vi "Channel_OFFSet.vi"(7 "Write?":bool, 8 "Error":errorcluster caption="错误输入（无错误）", 9 "Offset":dbl, 10 "Channel":u32, 11 "VISA resource name":refnum<visa-resource-name>) -> (0 "Error out":errorcluster, 2 "Offset out":dbl, 3 "VISA resource name out":refnum<visa-resource-name>)   [LabVIEW 2020]
doc: "屏幕中心显示的值"
panel:
  out "读取缓冲区":string
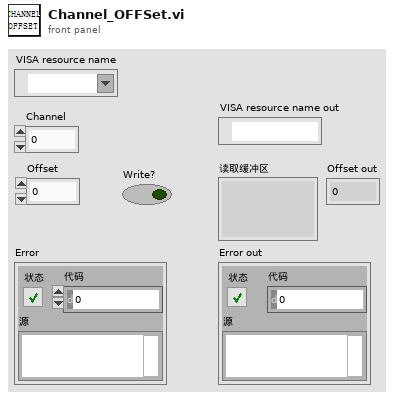
[diagram p1: front panel]
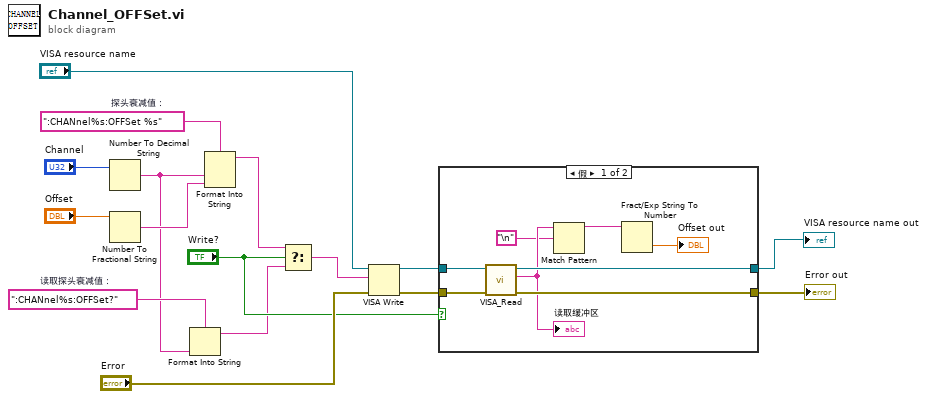
[diagram p0: block diagram]
diagram:
  w5 = ":CHANnel%s:OFFSet?"  # 读取探头衰减值：
  w9 = ":CHANnel%s:OFFSet %s"  # 探头衰减值：
  n1 = Number To Decimal String(number="Channel") -> (decimal integer string=w4:string)  [unwired: 1 in]
  n2 = Number To Fractional String(number="Offset") -> (F-format string=w7:string)  [unwired: 3 in]
  n3 = Format Into String(format string=w5, w4) -> (resulting string=w3:string)  [unwired: 2 in, 1 out]
  n4 = Format Into String(format string=w9, w4, w7) -> (resulting string=w6:string)  [unwired: 2 in, 1 out]
  n5 = Select(t=w6, s="Write?", f=w3) -> (s? t:f=w14:string)
  n6 = VISA Write(VISA resource name="VISA resource name", write buffer=w14, error in (no error)="Error") -> (VISA resource name out=w10:refnum<visa-resource-name>, error out=w12:errorcluster)  [unwired: 1 out]
  n7 = case shown="假" "Write?" {
    tunnel: w10 -> [w24 w26]
    tunnel: w12 -> [w23 w25]
    tunnel: [w21 w25] -> w11
    tunnel: [w22 w26] -> w1
    frame False {
      n8 = call "VISA_Read.vi"("Error"=w23, "VISA resource name"=w24) -> ("Error out"=w21:errorcluster, "读取缓冲区"=w20:string, "VISA resource name out"=w22:refnum<visa-resource-name>)  [unwired: 7 in]
      "读取缓冲区" <- w20
      n9 = Match Pattern(string=w20, regular expression="\n") -> (before substring=w18:string)  [unwired: 1 in, 3 out]
      n10 = Fract/Exp String To Number(string=w18) -> (number=→"Offset out":dbl)  [unwired: 3 in, 1 out]
    }
    frame True {
    }
  }
  "VISA resource name out" <- w1
  "Error out" <- w11
